vi "triplet-is pythagorean.vi"(8 "error in (no error)":errorcluster, 11 "(a, b, c) in":T1) -> (0 "error out":errorcluster, 3 "(a, b, c) out (duplicate)":T1)   [LabVIEW 2021, in "Project Euler.lvlib"]
uses:
  Project Euler.lvlib
  cluster-triplet.ctl
panel:
  out "T = this triplet is Pythagorean (a^2+b^2=c^2)":bool
  # "Development\ncontrols/indicators useful for development and testing, but which are not outputs of the VI"
  # "Input\nInputs to the VI"
  # "Output\nOutputs of the VI"
  # "Description\n\nBlank VI with error handling case. \n\nSummarize the use of this VI in this space."
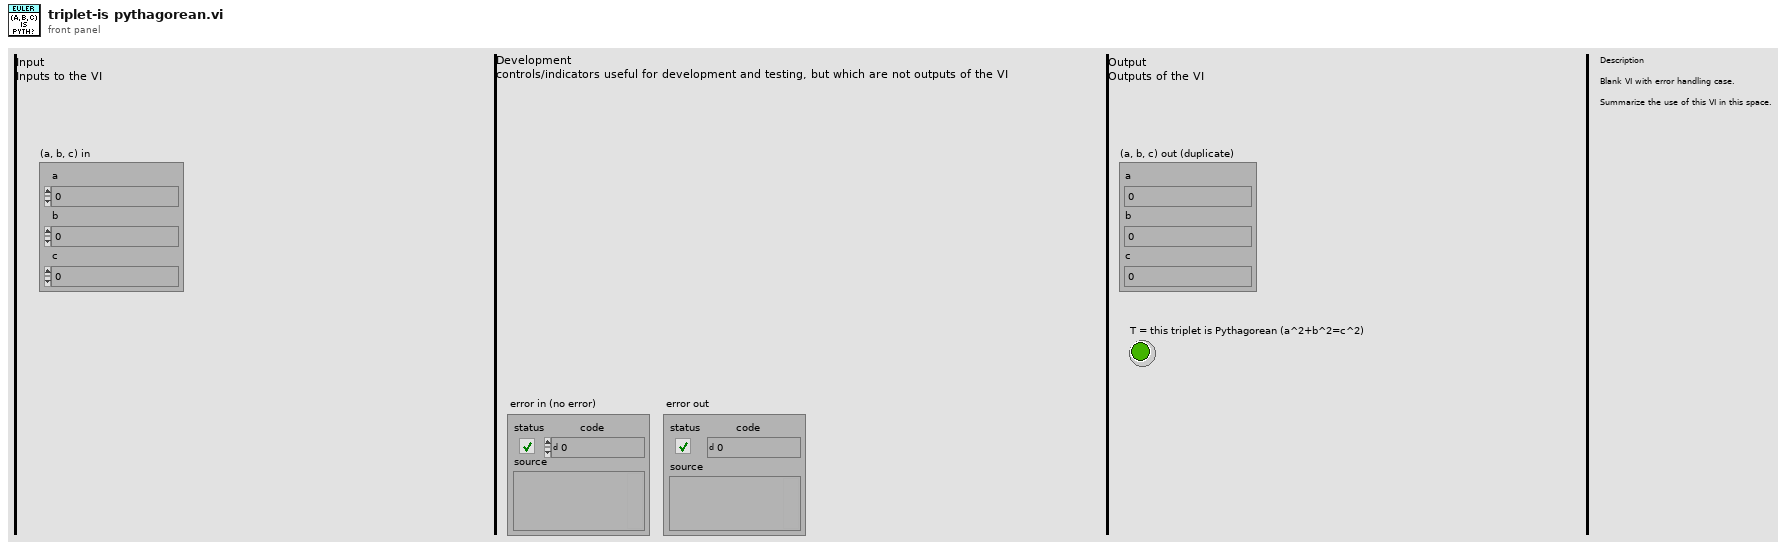
[diagram p1: front panel]
types:
  T1 = typedef "Project Euler.lvlib/cluster-triplet.ctl" = cluster{"a":i32, "b":i32, "c":i32}
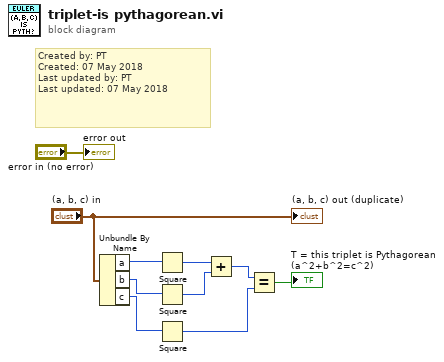
[diagram p0: block diagram]
diagram:
  # "Created by: PT\nCreated: 07 May 2018\nLast updated by: PT\nLast updated: 07 May 2018"
  n1 = Unbundle By Name("(a, b, c) in") -> ("a"=w8:i32, "b"=w7:i32, "c"=w6:i32)
  n2 = Square(x=w8) -> (x^2=w5:i32)
  n3 = Square(x=w7) -> (x^2=w4:i32)
  n4 = Square(x=w6) -> (x^2=w2:i32)
  n5 = Add(x=w5, y=w4) -> (x+y=w3:i32)
  n6 = Equal?(x=w3, y=w2) -> (x = y?=→"T = this triplet is Pythagorean (a^2+b^2=c^2)":bool)
  "error out" <- "error in (no error)"
  "(a, b, c) out (duplicate)" <- "(a, b, c) in"
